vi "Move Relative SubVi.vi"(2 "Horizontal Segments Parameters":T1(array[cluster]) {"Y rel dist" min=-100.0 max=100.0; "X rel dist" min=-100.0 max=100.0}, 3 "error in":errorcluster, 4 "reference in":refnum<k24>, 5 "Vertical Segments Parameters":T1(array[cluster]) {"Y rel dist" min=-100.0 max=100.0; "X rel dist" min=-100.0 max=100.0}) -> (0 "error in 2":errorcluster, 1 "reference out":refnum<k24>)   [LabVIEW 2017]
uses:
  Newport.XPS.CommandInterface
  Relative Move Enum.ctl
  Intermediate Relative Move Enum.ctl
  Inner Relaive Move Enum.ctl
  Inner Relative Move horizontal Enum.ctl
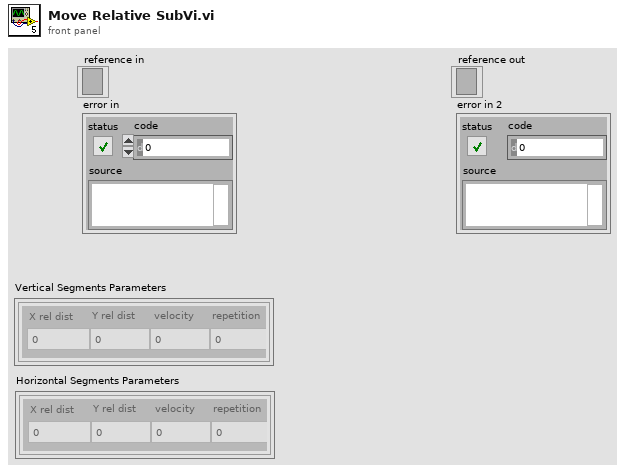
[diagram p1: front panel]
types:
  T1 = cluster{"X rel dist":dbl, "Y rel dist":dbl, "velocity":dbl, "repetition":u32}[]
  T2 = typedef "Relative Move Enum.ctl" = enum16{"Vertical Relative Motion", "Horizontal Relative Motion", "Stop Command"}
  T3 = typedef "Intermediate Relative Move Enum.ctl" = enum16{"Change Velocity", "Movment", "Stop Command"}
  T4 = enum16{"Wait Y", "Move Y", "Wait X", "Move X", "Stop Command"}
  T5 = typedef "Inner Relaive Move Enum.ctl" = enum16{"Wait Y", "Move Y", "Wait X", "Move X"}
  T6 = typedef "Inner Relative Move horizontal Enum.ctl" = enum16{"Wait Y", "Move Y", "Wait X", "Move X", "Stop Command"}
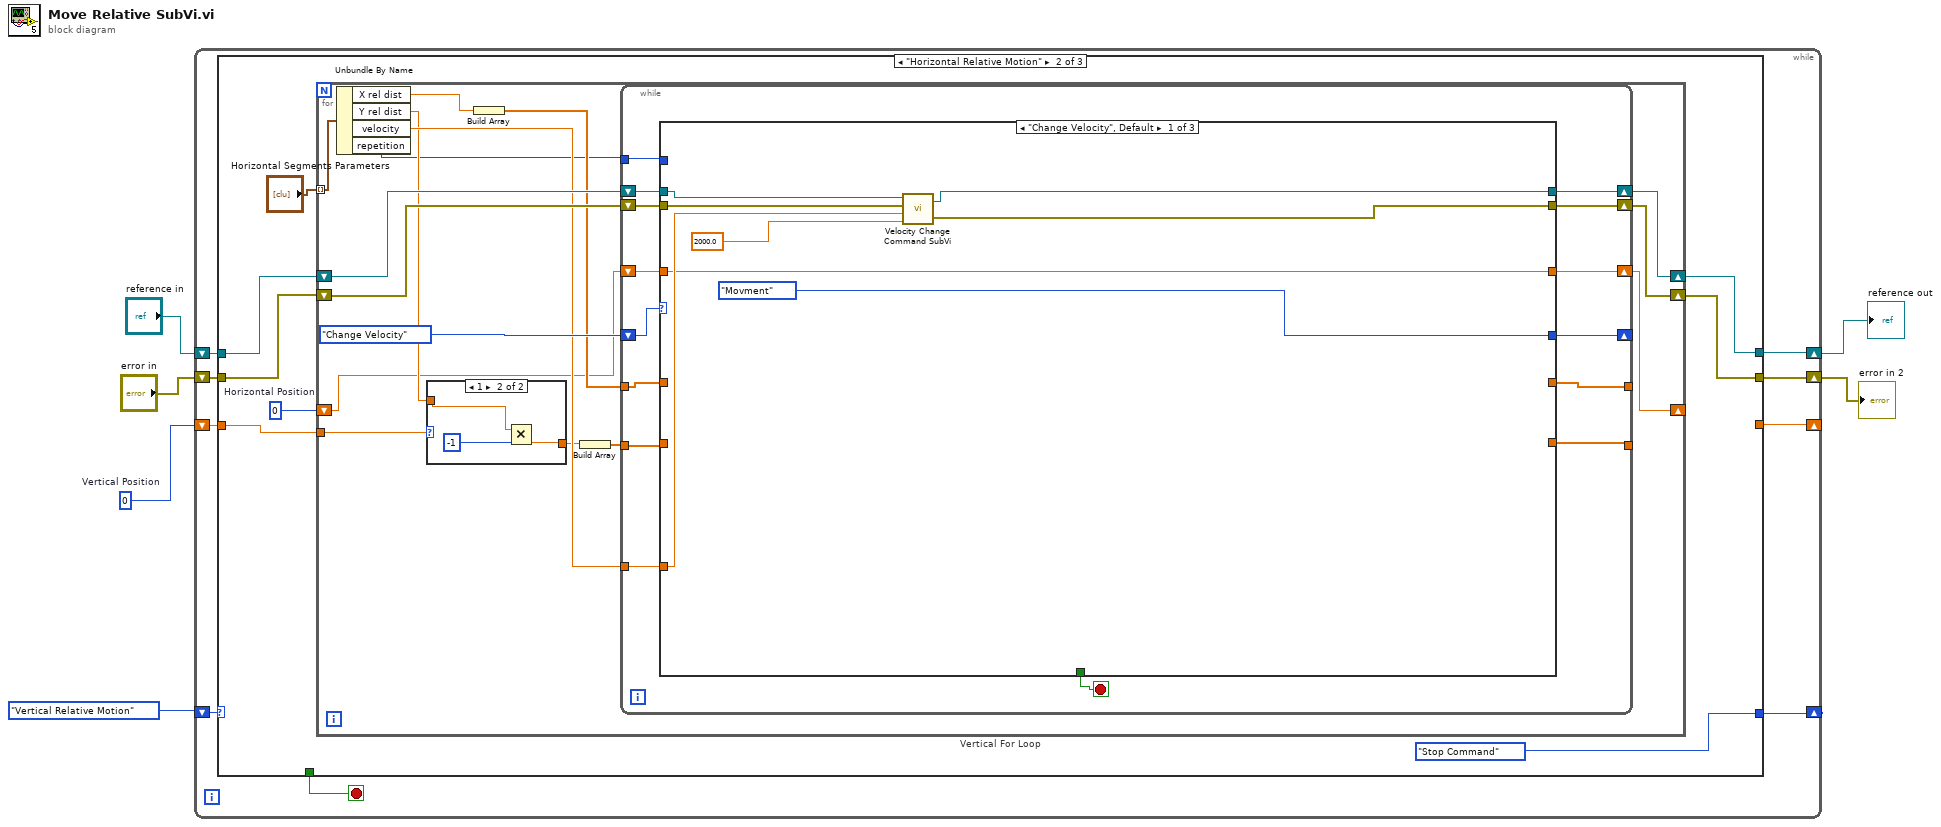
[diagram p0: block diagram]
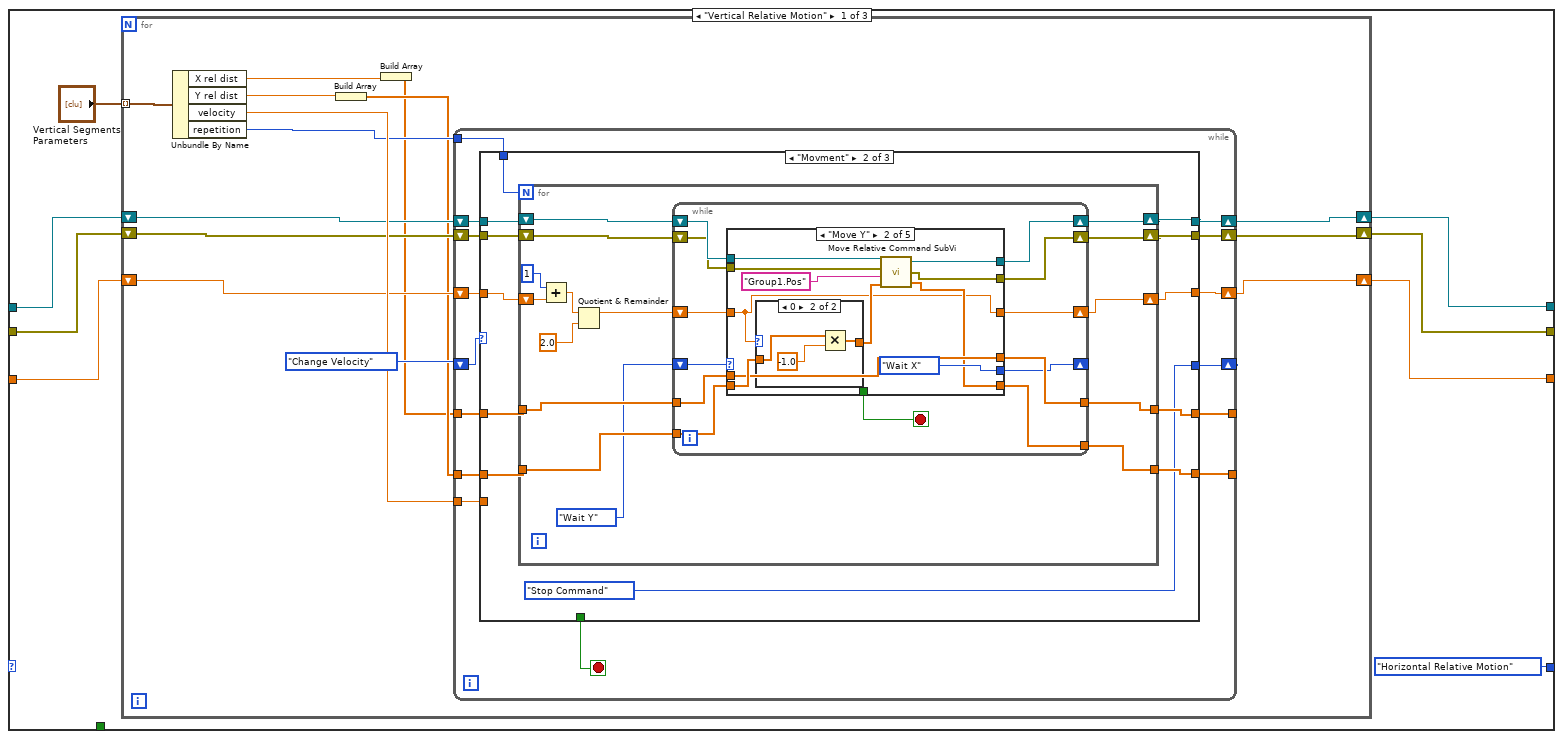
[diagram p2: hidden frame]
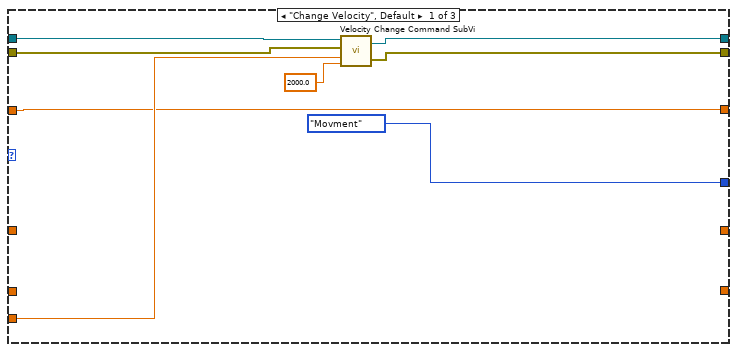
[diagram p3: hidden frame]
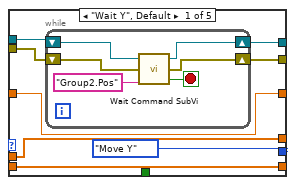
[diagram p4: hidden frame]
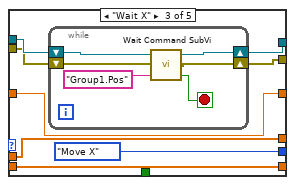
[diagram p6: hidden frame]
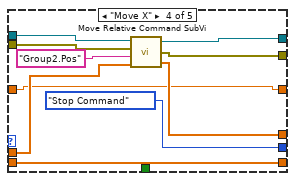
[diagram p7: hidden frame]
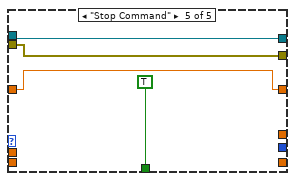
[diagram p8: hidden frame]
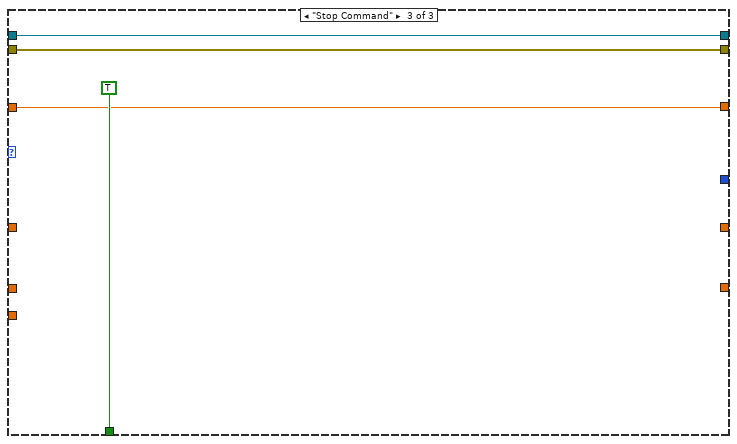
[diagram p9: hidden frame]
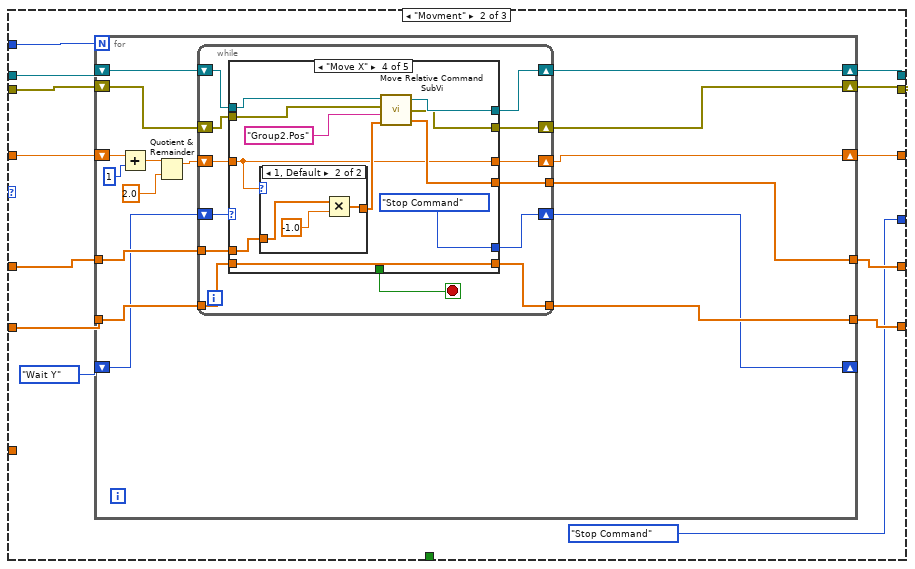
[diagram p10: hidden frame]
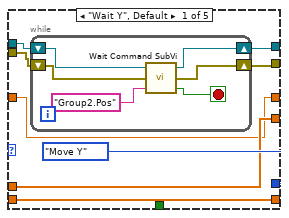
[diagram p11: hidden frame]
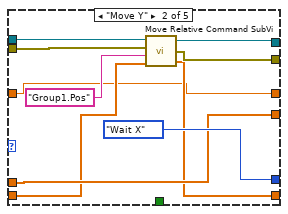
[diagram p12: hidden frame]
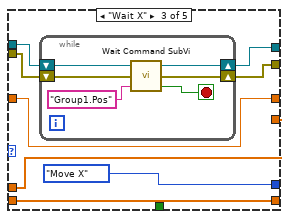
[diagram p13: hidden frame]
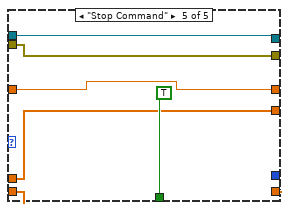
[diagram p15: hidden frame]
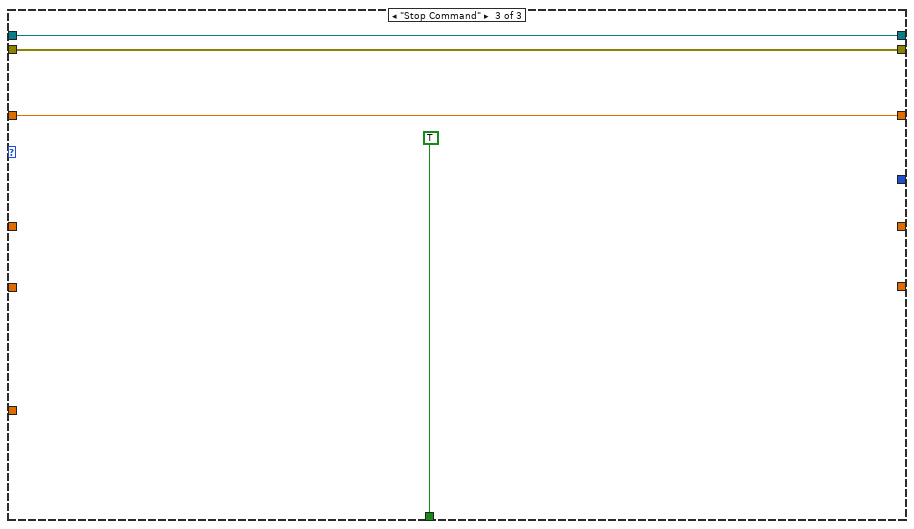
[diagram p16: hidden frame]
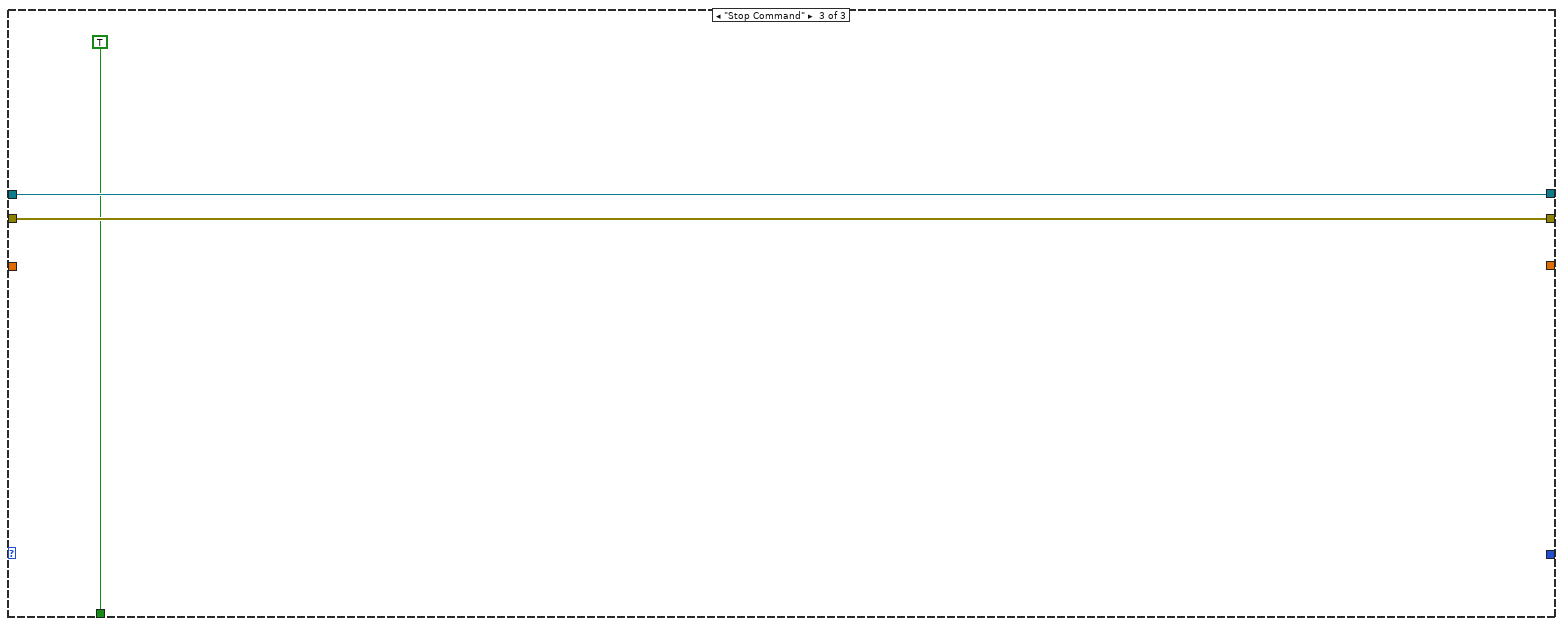
[diagram p18: hidden frame]
diagram:
  w2 = 0  # Vertical Position
  n1 = while {
    shift-right: [w14] -> _
    shift-left: Relative_Move_Enum."Vertical Relative Motion" -> [w15]
    shift-right: [w8] -> w4
    shift-left: "reference in" -> [w12]
    shift-right: [w9] -> w3
    shift-left: "error in" -> [w13]
    shift-right: [w10] -> _
    shift-left: w2 -> [w11]
    stop <- w7 stop-if-true
    n2 = case shown="\"Horizontal Relative Motion\"" w15 {
      tunnel: [Relative_Move_Enum."Horizontal Relative Motion" Relative_Move_Enum."Stop Command" _] -> w14
      tunnel: w13 -> [w23 w167 w319]
      tunnel: w12 -> [w22 w168 w320]
      tunnel: [w20 w166 w320] -> w8
      tunnel: w11 -> [w16 w169 _]
      tunnel: [w21 _ _] -> w10
      tunnel: [w19 w165 w319] -> w9
      tunnel: [_ _ TRUE] -> w7
      frame "Vertical Relative Motion" {
        n3 = for {
          tunnel: "Vertical Segments Parameters" -> [w37] mode=indexing
          shift-right: [w24] -> w21
          shift-left: w16 -> [w30]
          shift-right: [w27] -> w20
          shift-left: w22 -> [w33]
          shift-right: [w26] -> w19
          shift-left: w23 -> [w32]
          n4 = Unbundle By Name(w37) -> ("X rel dist"=w25:dbl, "Y rel dist"=w36:dbl, "velocity"=w34:dbl, "repetition"=w31:u32)
          n5 = Build Array(w36) -> (w29:dbl[])
          n6 = Build Array(w25) -> (w28:dbl[])
          n7 = while {
            shift-right: [w46] -> _
            shift-left: Intermediate_Relative_Move_Enum."Change Velocity" -> [w52]
            shift-right: [w48] -> w27
            shift-left: w33 -> [w50]
            shift-right: [w47] -> w26
            shift-left: w32 -> [w49]
            tunnel: w31 -> [w45]
            tunnel: w34 -> [w51]
            tunnel: w28 -> [w42]
            tunnel: [w41] -> _
            tunnel: w29 -> [w43]
            tunnel: [w40] -> _
            shift-right: [w38] -> w24
            shift-left: w30 -> [w44]
            stop <- w39 stop-if-true
            n8 = case shown="\"Movment\"" w52 {
              tunnel: w51 -> [w57 _ _]
              tunnel: w50 -> [w59 w71 w161]
              tunnel: w49 -> [w58 w70 w160]
              tunnel: [w55 w64 w161] -> w48
              tunnel: [w54 w63 w160] -> w47
              tunnel: [Intermediate_Relative_Move_Enum."Movment" Intermediate_Relative_Move_Enum."Stop Command" _] -> w46
              tunnel: w45 -> [_ w72 _]
              tunnel: w44 -> [w53 w69 w158]
              tunnel: w43 -> [_ w68 _]
              tunnel: w42 -> [_ w67 _]
              tunnel: [_ w66 _] -> w41
              tunnel: [_ w65 _] -> w40
              tunnel: [_ _ TRUE] -> w39
              tunnel: [w53 w61 w158] -> w38
              frame "Change Velocity", Default {
                n9 = call "Velocity Change Command SubVi.vi"("Acceleration"=2000.0, "Velocity"=w57, "error in"=w58, "reference in"=w59) -> ("error out"=w54:errorcluster, "reference out"=w55:refnum<k24>)
              }
              frame "Movment" {
                n10 = for {
                  N: w72 -> [_]
                  shift-right: [w79] -> w63
                  shift-left: w70 -> [w81]
                  shift-right: [w80] -> w64
                  shift-left: w71 -> [w82]
                  tunnel: w67 -> [w77]
                  tunnel: [w76] -> w66
                  tunnel: w68 -> [w83]
                  tunnel: [w78] -> w65
                  shift-right: [w73] -> w61
                  shift-left: w69 -> [w84]
                  n11 = Add(x=1, y=w84) -> (x+y=w87:dbl)
                  n12 = Quotient & Remainder(x=w87, y=2.0) -> (x-y*floor(x/y)=w86:dbl)  [unwired: 1 out]
                  n13 = while {
                    shift-right: [w91] -> w80
                    shift-left: w82 -> [w98]
                    shift-right: [w90] -> w79
                    shift-left: w81 -> [w97]
                    shift-right: [w92] -> _
                    shift-left: T4."Wait Y" -> [w93]
                    tunnel: w77 -> [w95]
                    tunnel: [w94] -> w76
                    tunnel: w83 -> [w99]
                    tunnel: [w96] -> w78
                    shift-right: [w88] -> w73
                    shift-left: w86 -> [w100]
                    stop <- w89 stop-if-true
                    n14 = case shown="\"Move Y\"" w93 {
                      tunnel: [Inner_Relaive_Move_Enum."Move Y" T4."Wait X" Inner_Relaive_Move_Enum."Move X" T4."Stop Command" _] -> w92
                      tunnel: w100 -> [w101 w115 w130 w144 w154]
                      tunnel: w99 -> [w106 w125 w135 w153 _]
                      tunnel: w98 -> [w104 w122 w134 w152 w157]
                      tunnel: w97 -> [w105 w121 w132 w151 w156]
                      tunnel: [w106 w117 w135 w153 _] -> w96
                      tunnel: w95 -> [w107 w123 w136 w147 _]
                      tunnel: [w107 w123 w136 w146 _] -> w94
                      tunnel: [w103 w119 w133 w150 w157] -> w91
                      tunnel: [w102 w118 w131 w149 w156] -> w90
                      tunnel: [_ _ _ _ TRUE] -> w89
                      tunnel: [w101 w115 w130 w144 w154] -> w88
                      frame "Wait Y", Default {
                        n15 = while {
                          shift-right: [w113] -> w102
                          shift-left: w105 -> [w110]
                          shift-right: [w114] -> w103
                          shift-left: w104 -> [w109]
                          stop <- w112 stop-if-true
                          n16 = call "Wait Command SubVi.vi"("GroupName"="Group2.Pos", "error in"=w110, "reference in"=w109) -> ("Is Stop"=w112:bool, "error out"=w113:errorcluster, "reference out"=w114:refnum<k24>)
                        }
                      }
                      frame "Move Y" {
                        n17 = case shown="0" w115 {
                          tunnel: w125 -> [w126 w127]
                          tunnel: [w126 w128] -> w116
                          frame 1, Default {
                          }
                          frame 0 {
                            n18 = Multiply(x=w127, y=-1.0) -> (x*y=w128:dbl[])
                          }
                        }
                        n19 = call "Move Relative Command SubVi.vi"("TargetDisplacement in"=w116, "GroupName"="Group1.Pos", "error in"=w121, "reference in"=w122) -> ("TargetDisplacement out"=w117:dbl[], "error out"=w118:errorcluster, "reference out"=w119:refnum<k24>)
                      }
                      frame "Wait X" {
                        n20 = while {
                          shift-right: [w140] -> w133
                          shift-left: w134 -> [w143]
                          shift-right: [w139] -> w131
                          shift-left: w132 -> [w142]
                          stop <- w138 stop-if-true
                          n21 = call "Wait Command SubVi.vi"("GroupName"="Group1.Pos", "error in"=w142, "reference in"=w143) -> ("Is Stop"=w138:bool, "error out"=w139:errorcluster, "reference out"=w140:refnum<k24>)
                        }
                      }
                      frame "Move X" {
                        n22 = call "Move Relative Command SubVi.vi"("TargetDisplacement in"=w147, "GroupName"="Group2.Pos", "error in"=w151, "reference in"=w152) -> ("TargetDisplacement out"=w146:dbl[], "error out"=w149:errorcluster, "reference out"=w150:refnum<k24>)
                      }
                      frame "Stop Command" {
                      }
                    }
                  }
                }
              }
              frame "Stop Command" {
              }
            }
          }
        }
      }
      frame "Horizontal Relative Motion" {
        w162 = 0  # Horizontal Position
        n23 = for "Vertical For Loop" {
          tunnel: "Horizontal Segments Parameters" -> [w185] mode=indexing
          tunnel: w169 -> [w170]
          shift-right: [w180] -> w166
          shift-left: w168 -> [w183]
          shift-right: [w179] -> w165
          shift-left: w167 -> [w182]
          shift-right: [w171] -> _
          shift-left: w162 -> [w172]
          n24 = Unbundle By Name(w185) -> ("X rel dist"=w175:dbl, "Y rel dist"=w178:dbl, "velocity"=w181:dbl, "repetition"=w173:u32)
          n25 = case shown="1" w170 {
            tunnel: [w314 w317] -> w177
            tunnel: w178 -> [w314 w315]
            frame 0, Default {
            }
            frame 1 {
              n26 = Multiply(x=w315, y=-1) -> (x*y=w317:dbl)
            }
          }
          n27 = Build Array(w175) -> (w174:dbl[])
          n28 = Build Array(w177) -> (w176:dbl[])
          n29 = while {
            shift-right: [w194] -> _
            shift-left: Intermediate_Relative_Move_Enum."Change Velocity" -> [w200]
            shift-right: [w196] -> w180
            shift-left: w183 -> [w198]
            shift-right: [w195] -> w179
            shift-left: w182 -> [w197]
            tunnel: w181 -> [w199]
            tunnel: w173 -> [w189]
            tunnel: w174 -> [w192]
            tunnel: [w191] -> _
            tunnel: w176 -> [w193]
            tunnel: [w190] -> _
            shift-right: [w186] -> w171
            shift-left: w172 -> [w187]
            stop <- w188 stop-if-true
            n30 = case shown="\"Change Velocity\", Default" w200 {
              tunnel: w199 -> [w205 _ _]
              tunnel: w198 -> [w207 w221 w313]
              tunnel: w197 -> [w206 w220 w312]
              tunnel: [w203 w215 w313] -> w196
              tunnel: [w202 w214 w312] -> w195
              tunnel: [Intermediate_Relative_Move_Enum."Movment" Intermediate_Relative_Move_Enum."Stop Command" _] -> w194
              tunnel: w193 -> [_ w219 _]
              tunnel: w192 -> [_ w218 _]
              tunnel: [_ w217 _] -> w191
              tunnel: [_ w216 _] -> w190
              tunnel: w189 -> [_ w212 _]
              tunnel: [_ _ TRUE] -> w188
              tunnel: w187 -> [w201 w210 w310]
              tunnel: [w201 w209 w310] -> w186
              frame "Change Velocity", Default {
                n31 = call "Velocity Change Command SubVi.vi"("Acceleration"=2000.0, "Velocity"=w205, "error in"=w206, "reference in"=w207) -> ("error out"=w202:errorcluster, "reference out"=w203:refnum<k24>)
              }
              frame "Movment" {
                n32 = for {
                  N: w212 -> [_]
                  shift-right: [w231] -> w214
                  shift-left: w220 -> [w233]
                  shift-right: [w232] -> w215
                  shift-left: w221 -> [w234]
                  shift-right: [w226] -> _
                  shift-left: Inner_Relative_Move_horizontal_Enum."Wait Y" -> [w227]
                  tunnel: w218 -> [w229]
                  tunnel: [w228] -> w217
                  tunnel: w219 -> [w235]
                  tunnel: [w230] -> w216
                  shift-right: [w222] -> w209
                  shift-left: w210 -> [w225]
                  n33 = Add(x=w225, y=1) -> (x+y=w224:dbl)
                  n34 = Quotient & Remainder(x=w224, y=2.0) -> (x-y*floor(x/y)=w237:dbl)  [unwired: 1 out]
                  n35 = while {
                    tunnel: w235 -> [w249]
                    tunnel: [w244] -> w230
                    tunnel: w229 -> [w243]
                    tunnel: [w242] -> w228
                    shift-right: [w246] -> w232
                    shift-left: w234 -> [w248]
                    shift-right: [w245] -> w231
                    shift-left: w233 -> [w247]
                    shift-right: [w240] -> w226
                    shift-left: w227 -> [w241]
                    shift-right: [w238] -> w222
                    shift-left: w237 -> [w250]
                    stop <- w239 stop-if-true
                    n36 = case shown="\"Move X\"" w241 {
                      tunnel: [Inner_Relative_Move_horizontal_Enum."Move Y" Inner_Relative_Move_horizontal_Enum."Wait X" Inner_Relative_Move_horizontal_Enum."Move X" Inner_Relative_Move_horizontal_Enum."Stop Command" _] -> w240
                      tunnel: w250 -> [w251 w265 w275 w289 w304]
                      tunnel: w249 -> [w256 w269 w281 w297 w307]
                      tunnel: w248 -> [w255 w272 w279 w296 w306]
                      tunnel: w247 -> [w254 w271 w278 w295 w305]
                      tunnel: [w253 w268 w277 w291 w306] -> w246
                      tunnel: [w252 w267 w276 w290 w305] -> w245
                      tunnel: [w256 w266 w281 w297 w307] -> w244
                      tunnel: w243 -> [w257 w273 w280 w298 w308]
                      tunnel: [w257 w273 w280 w292 w308] -> w242
                      tunnel: [_ _ _ _ TRUE] -> w239
                      tunnel: [w251 w265 w275 w289 w304] -> w238
                      frame "Wait Y", Default {
                        n37 = while {
                          shift-right: [w260] -> w252
                          shift-left: w254 -> [w263]
                          shift-right: [w261] -> w253
                          shift-left: w255 -> [w264]
                          stop <- w259 stop-if-true
                          n38 = call "Wait Command SubVi.vi"("GroupName"="Group2.Pos", "error in"=w263, "reference in"=w264) -> ("Is Stop"=w259:bool, "error out"=w260:errorcluster, "reference out"=w261:refnum<k24>)
                        }
                      }
                      frame "Move Y" {
                        n39 = call "Move Relative Command SubVi.vi"("TargetDisplacement in"=w269, "GroupName"="Group1.Pos", "error in"=w271, "reference in"=w272) -> ("TargetDisplacement out"=w266:dbl[], "error out"=w267:errorcluster, "reference out"=w268:refnum<k24>)
                      }
                      frame "Wait X" {
                        n40 = while {
                          shift-right: [w285] -> w277
                          shift-left: w279 -> [w288]
                          shift-right: [w284] -> w276
                          shift-left: w278 -> [w287]
                          stop <- w283 stop-if-true
                          n41 = call "Wait Command SubVi.vi"("GroupName"="Group1.Pos", "error in"=w287, "reference in"=w288) -> ("Is Stop"=w283:bool, "error out"=w284:errorcluster, "reference out"=w285:refnum<k24>)
                        }
                      }
                      frame "Move X" {
                        n42 = case shown="1, Default" w289 {
                          tunnel: w298 -> [w300 w301]
                          tunnel: [w300 w302] -> w293
                          frame 0 {
                          }
                          frame 1, Default {
                            n43 = Multiply(x=w301, y=-1.0) -> (x*y=w302:dbl[])
                          }
                        }
                        n44 = call "Move Relative Command SubVi.vi"("TargetDisplacement in"=w293, "GroupName"="Group2.Pos", "error in"=w295, "reference in"=w296) -> ("TargetDisplacement out"=w292:dbl[], "error out"=w290:errorcluster, "reference out"=w291:refnum<k24>)
                      }
                      frame "Stop Command" {
                      }
                    }
                  }
                }
              }
              frame "Stop Command" {
              }
            }
          }
        }
      }
      frame "Stop Command" {
      }
    }
  }
  "reference out" <- w4
  "error in 2" <- w3
